vi "Heater.vi"(0 "Heater in":refnum<class "Heater.lvclass">, 1 "Z_ASetState":T4, 2 "ALRs":bool[](array[boolean])=[FALSE, FALSE, FALSE], 5 "ZY_control":T3 {"Y_H" step=1.0; "SP" step=0.01 format="%.2f"}, 7 "PV":dbl step=0.01 format="%.2f", 9 "PV state":T2, 11 "error in (no error)":errorcluster, 12 "ALR_Status":T1[](array[typedef]), 13 "DI":bool[](array[boolean])) -> (4 "Heater out":refnum<class "Heater.lvclass">, 6 "ZY_State":T6 {"Y"."Y_Set" format="%.2f"; "Y"."SP" step=0.01 format="%.2f"; "Y"."Y" format="%.2f"; "Y"."PV" step=0.01 format="%.2f"; "Y"."SP_Set" step=0.01 format="%.2f"}, 8 "Y":dbl format="%.2f", 10 "YB":bool[](array[boolean]), 14 "ALR_ON":bool[](array[boolean]), 15 "error out":errorcluster)   [LabVIEW 2019, in "Heating.lvlib" / "Heater.lvclass"]
uses:
  Heater.lvclass
  ctl/Z_State.ctl
  ctl/ZY_state_short.ctl
  ctl/Z.ctl
  ctl/Z_source.ctl
  ctl/ZM_State.ctl
  ctl/Y_short.ctl
  ctl/Y_source.ctl
  ctl/Y_state.ctl
  Inputs/Ctl/Parameter State short.ctl
  Alarms/Ctl/ALR_Status_short.ctl
  ctl/ZY_control.ctl
  Heater.lvclass/Heater.ctl
  REG/HE_reg.lvclass/HE_reg.ctl
  Reg/PID/PID SP Limiter/PID SP Limiter.lvclass/PID SP Limiter.ctl
  HE_state.lvclass/HE_state.ctl
  ZM_state/HE_ZM_state.lvclass/HE_ZM_state.ctl
  Z_state/HE_Z_state.lvclass/HE_Z_state.ctl
  Sequence/State/State.lvclass/State.ctl
  Reg/PID/PID Output Rate Limiter/PID Output Rate Limiter.lvclass/PID Output Rate Limiter.ctl
  Reg/PID/PID Timing Estimation/PID Timing Estimation.lvclass/PID Timing Estimation.ctl
  Reg/PID/PID_OL_AM/PID_OL_AM.lvclass/PID_OL_AM.ctl
  Transform/Impulsator.lvclass/Impulsator.ctl
  Z_switch_heating.vi
  ZM_state/Read ZM_State.vi
  Z_state/Z_state.vi
  Z_state/Read T.vi
  Z_state/Read Z_State.vi
  ZM_state/ZM_state.vi
  ZM_state/Read T.vi
  Y_switch_heating.vi
  Reg/PID/PID SP Limiter/PID SP Limiter.vi
  Reg/PID/PID_OL_AM/PID_OL_AM.vi
  Transform/ImpulsatorC.vi
  Reg/PID/PID_OL_AM/Write output H.vi
  Reg/PID/PID SP Limiter/Read T.vi
  ZM_state/Write T start_stop.vi
  Read ZM_state.vi
  Write ZM_state.vi
  REG/Read PID SP Lim.vi
  Reg/PID/PID SP Limiter/Read End.vi
  Sequence/State/Read T (ms).vi
  Reg/PID/PID Output Rate Limiter/PID Output Rate Limiter.vi
  Reg/PID/PID Output Rate Limiter/Write output rate.vi
  Reg/PID/PID Timing Estimation/PID Timing Estimation.vi
  Reg/PID/PID Output Rate Limiter/Read output.vi
  Z_state/HE_Z_state.lvclass
  D:/my_projects/projects/Algorithms/Labview/19/Sequence/State/State.lvclass
  ZM_state/HE_ZM_state.lvclass
  Reg/PID/PID SP Limiter/PID SP Limiter.lvclass
  D:/my_projects/projects/Algorithms/Labview/19/Reg/PID/PID Output Rate Limiter/PID Output Rate Limiter.lvclass
  Reg/PID/PID Output Rate Limiter/PID Output Rate Limiter.lvclass
  D:/my_projects/projects/Algorithms/Labview/19/Reg/PID/PID Timing Estimation/PID Timing Estimation.lvclass
  REG/HE_reg.lvclass
  D:/my_projects/projects/Algorithms/Labview/19/Reg/PID/PID_OL_AM/PID_OL_AM.lvclass
  Reg/PID/PID_OL_AM/PID_OL_AM.lvclass
  Sequence/State/Step.vi
  Heating.lvlib
  Alarms/Alarms.lvlib
  Inputs/Inputs.lvlib
  HE_state.lvclass
panel:
  # "0 bit - Alarm level 1\n1 bit - Alarm level 2\n2 bit - Alarm level 3"
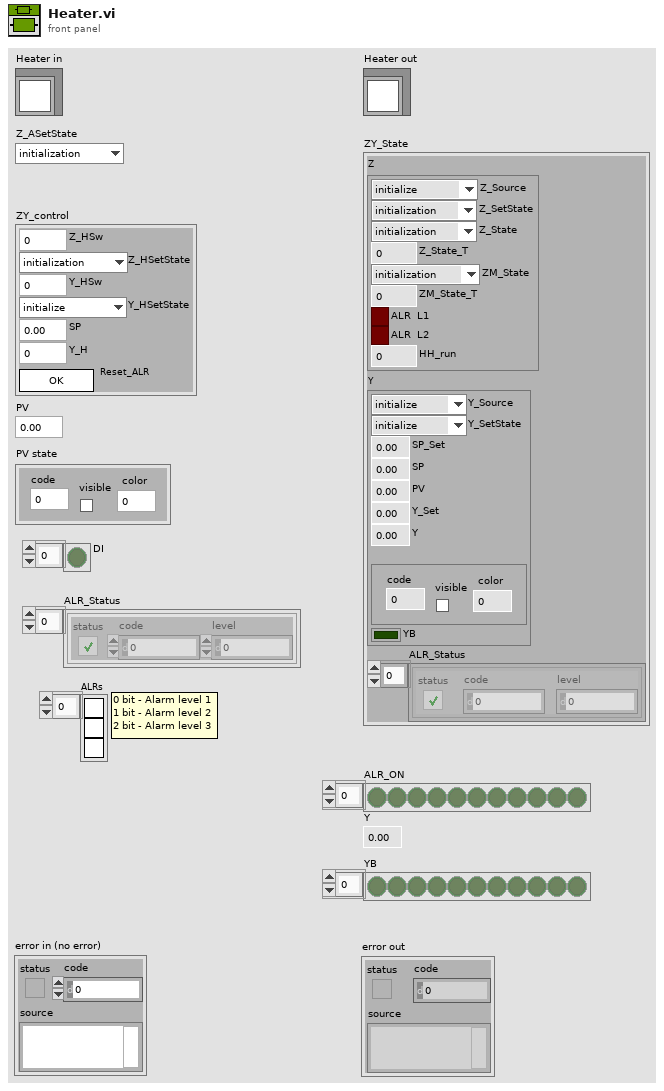
[diagram p1: front panel]
types:
  T1 = typedef "Alarms.lvlib/ALR_Status_short.ctl" = cluster{"status":bool, "code":i32, "level":i32}
  T2 = typedef "Inputs.lvlib/Parameter State short.ctl" = cluster{"code":i32, "visible":bool, "color":u32}
  T3 = typedef "Heating.lvlib/ZY_control.ctl" = cluster{"Z_HSw":u8, "Z_HSetState":T4, "Y_HSw":u8, "Y_HSetState":T5, "SP":dbl, "Y_H":dbl, "Reset_ALR":bool}
  T4 = typedef "Heating.lvlib/Z_State.ctl" = enum8{"initialization", "alarm", "disabled", "not ready", "stop ready", "reserv", "switched off", "reserv2", "switched on", "check", "on min", "decrease out", "on", "increase out", "on max"}
  T5 = typedef "Heating.lvlib/Y_state.ctl" = enum8{"initialize", "alarm", "min", "stop", "hand", "auto", "max"}
  T6 = typedef "Heating.lvlib/ZY_state_short.ctl" = cluster{"Z":T7, "Y":T10, "ALR_Status":T1[]}
  T7 = typedef "Heating.lvlib/Z.ctl" = cluster{"Z_Source":T8, "Z_SetState":T4, "Z_State":T4, "Z_State_T":u32, "ZM_State":T9, "ZM_State_T":u32, "ALR  L1":bool, "ALR  L2":bool, "HH_run":u64}
  T8 = typedef "Heating.lvlib/Z_source.ctl" = enum8{"initialize", "local disabled", "local hand", "hand", "auto", "dist"}
  T9 = typedef "Heating.lvlib/ZM_State.ctl" = enum8{"initialization", "stop", "start_cmd", "contactor_on_cmd", "heating", "on", "stop_cmd", "power_down", "contactor_off_cmd", "cooling", "restart_delay"}
  T10 = typedef "Heating.lvlib/Y_short.ctl" = cluster{"Y_Source":T11, "Y_SetState":T5, "SP_Set":dbl, "SP":dbl, "PV":dbl, "Y_Set":dbl, "Y":dbl, "Y_State":T2, "YB":bool}
  T11 = typedef "Heating.lvlib/Y_source.ctl" = enum8{"initialize", "local disabled", "local hand", "hand", "auto", "dist"}
  T12 = typedef "Heating.lvlib/Z_control.ctl" = cluster{"Z_HSw":u8, "Z_HSetState":T4, "Z_ASetState":T4, "Z_DSetState":T4}
  T13 = typedef "Heating.lvlib/Y_control.ctl" = cluster{"Y_HSw":u8, "Y_HSetState":T5, "Y_ASetState":T5, "Y_DSetState":T5}
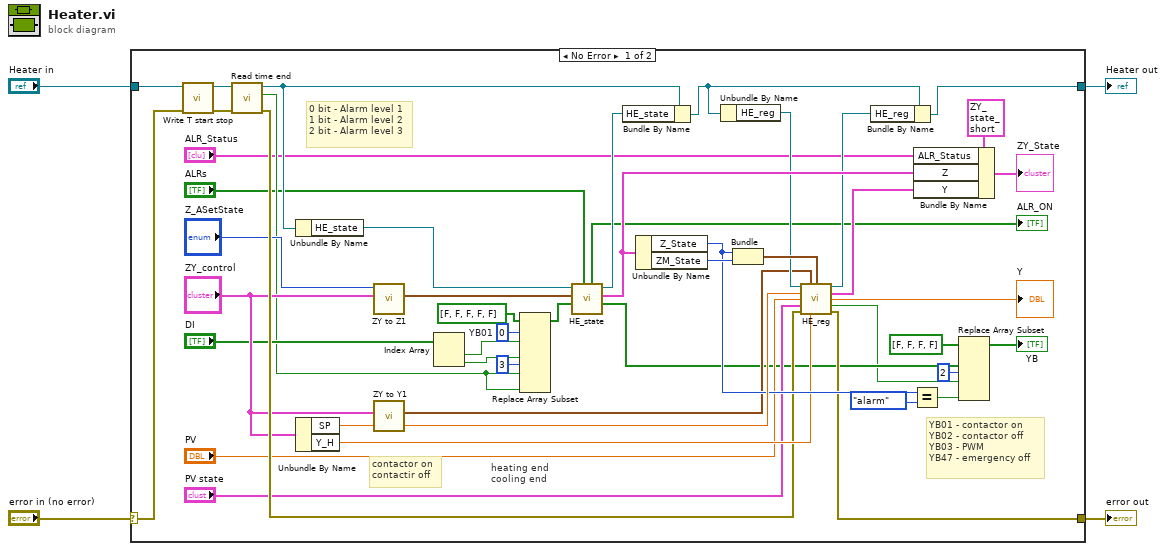
[diagram p0: block diagram]
diagram:
  n1 = case shown="No Error" "error in (no error)" {
    selector: "error in (no error)" -> [w29 w53]
    tunnel: [w27 w53] -> w3
    tunnel: [w30 w52] -> w1
    tunnel: "Heater in" -> [w24 w52]
    frame No Error {
      w51 = 0  # YB01
      # "0 bit - Alarm level 1\n1 bit - Alarm level 2\n2 bit - Alarm level 3"
      # "YB01 - contactor on\nYB02 - contactor off\nYB03 - PWM\nYB47 - emergency off"
      # "contactor on\ncontactir off"
      # "heating end\ncooling end"
      n2 = call "Write T start stop.vi"("error in (no error)"=w29, "Heater in"=w24) -> ("error out"=w34:errorcluster, "Heater out"=w36:refnum<class "Heater.lvclass">)  [unwired: 8 in]
      n3 = call "Read time end.vi"("error in (no error)"=w34, "Heater in"=w36) -> ("error out"=w28:errorcluster, "End"=w8:bool, "Heater out"=w25:refnum<class "Heater.lvclass">)  [unwired: 7 in]
      n4 = Unbundle By Name(w25) -> ("HE_state"=w10:refnum<class "HE_state.lvclass">)
      n5 = Unbundle By Name("ZY_control") -> ("SP"=w43:dbl, "Y_H"=w37:dbl)
      n6 = call "ZY to Z1.vi"("ZY_control"="ZY_control", "Z_ASetState"="Z_ASetState") -> ("Z_control"=w21:T12)  [unwired: 9 in]
      n7 = call "ZY to Y1.vi"("ZY_control"="ZY_control") -> ("Y"=w19:T13)  [unwired: 10 in]
      n8 = Index Array ("YB01")(array="DI") -> (element #1=w38:bool, element #2=w7:bool)  [unwired: 2 in]
      n9 = Replace Array Subset(array=bool[] [FALSE, FALSE, FALSE, FALSE, FALSE] ("XB"), new element #1=w38, index #1=w51, new element #2=w7, new element #3=w8, index #3=3 ("he end"), new element #4=w8) -> (w39:bool[])  [unwired: 2 in]
      n10 = call "HE_state.vi"("Alarm"="ALRs", "XB"=w39, "Z_control"=w21, "HE1_state_in"=w10) -> ("YB"=w16:bool[], "Z"=w46:T7, "HE1_state_out"=w35:refnum<class "HE_state.lvclass">, "ALR_ON"=→"ALR_ON":bool[])  [unwired: 4 in]
      n11 = Bundle By Name(cluster=w25, "HE_state"=w35) -> (w31:refnum<class "Heater.lvclass">)
      n12 = Unbundle By Name(w46) -> ("Z_State"=w40:T4, "ZM_State"=w48:T9)
      n13 = Unbundle By Name(w31) -> ("HE_reg"=w33:refnum<class "HE_reg.lvclass">)
      n14 = Bundle("Z_State"=w40, "ZM_State"=w48) -> (w47:cluster{"Z_State":T4, "ZM_State":T9})  [unwired: 1 in]
      n15 = call "HE_reg.vi"("HE_reg in"=w33, "Y"=w19, "Z"=w47, "SP"=w43, "PV"="PV", "PV_State"="PV state", "error in (no error)"=w28, "Y_H"=w37) -> ("HE_reg out"=w32:refnum<class "HE_reg.lvclass">, "Y_State"=w45:T10, "Y"=→"Y":dbl, "YB"=w15:bool, "error out"=w27:errorcluster)  [unwired: 3 in]
      n16 = Bundle By Name(cluster=w31, "HE_reg"=w32) -> (w30:refnum<class "Heater.lvclass">)
      n17 = Equal?(x=w40, y=Z_State."alarm" ("Z_State")) -> (x = y?=w12:bool)
      n18 = Bundle By Name(cluster=T6 {"Z"={"Z_Source"=enum."local disabled", "Z_SetState"=enum."on", "Z_State"=enum."alarm", "Z_State_T"=0, "ZM_State"=enum."initialization", "ZM_State_T"=0, "ALR  L1"=FALSE, "ALR  L2"=FALSE, "HH_run"=0}, "Y"={"Y_Source"=enum."local disabled", "Y_SetState"=enum."auto", "SP_Set"=0.0, "SP"=0.0, "PV"=0.0, "Y_Set"=0.0, "Y"=0.0, "Y_State"={"code"=0, "visible"=FALSE, "color"=0}, "YB"=FALSE}, "ALR_Status"=[]} ("ZY_State"), "ALR_Status"="ALR_Status", "Z"=w46, "Y"=w45) -> (→"ZY_State":T6)
      n19 = Replace Array Subset(array=bool[] [FALSE, FALSE, FALSE, FALSE], new element #1=w16, new element #2=w15, index #2=2 ("index"), new element #3=w12) -> (→"YB":bool[])  [unwired: 2 in]
    }
    frame Error {
    }
  }
  "error out" <- w3
  "Heater out" <- w1
